vi "System Timing Test.vi"() -> ()   [LabVIEW 2020]
uses:
  e41e6262-df0e-46e3-b5d9-5448b0aad18a.vi
  71bacbc6-81ed-4225-8d97-44bb9760859f.vi
  57dc439b-a836-43f6-a4ee-51e2563579e4.vi
  <vilib>/Utility/High Resolution Relative Seconds.vi
  <vilib>/Analysis/NI_AALPro.lvlib
  <vilib>/gmath/NI_Gmath.lvlib
panel:
  out "Waveform Graph":dbl[](graph)
  out "median 3":dbl format="%.3f ms"
  out "timing 3":T1(graph)
  out "median 2":dbl format="%.3f ms"
  out "timing 2":T1(graph)
  out "median":dbl format="%.3f ms"
  out "timing":T1(graph)
  in  "repeats":i32=1800
  in  "milliseconds to wait":u32=990
  out "Iteration":i32
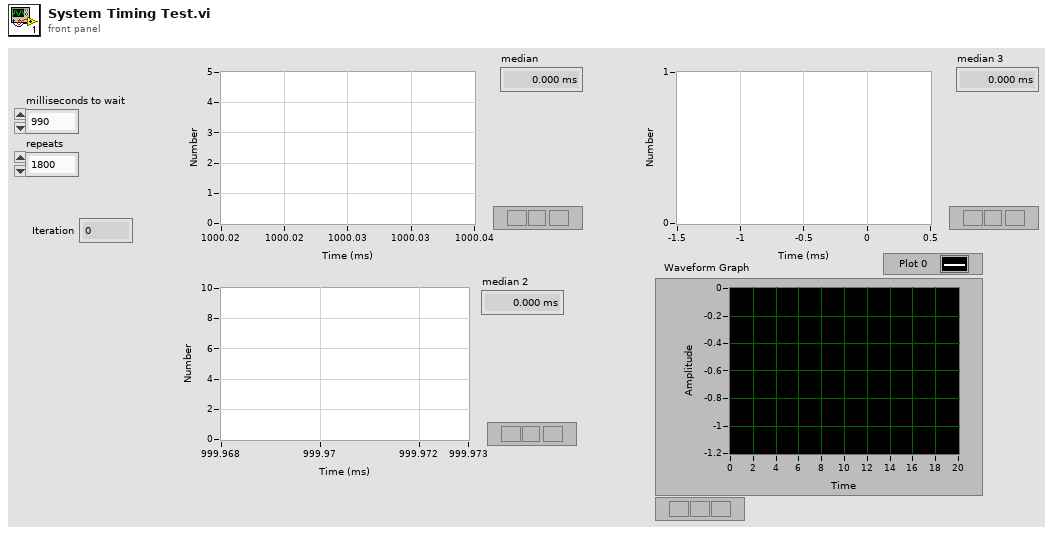
[diagram p1: front panel]
types:
  T1 = cluster{"X Values":dbl[], "Histogram: h(x)":i32[]}
  T2 = enum16{"arithmetic", "geometric", "harmonic", "trimmed", "median"}
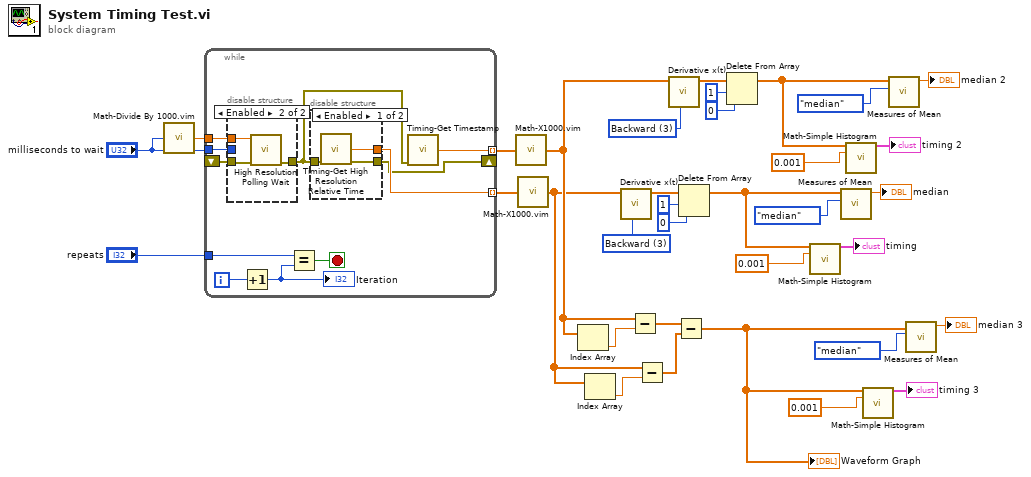
[diagram p0: block diagram]
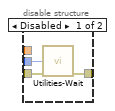
[diagram p2: hidden frame]
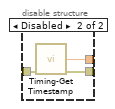
[diagram p3: hidden frame]
diagram:
  w20 = u16 3 items=["2nd Order Central", "4th Order Central", "Forward", "Backward"] ("method")
  w32 = u16 3 items=["2nd Order Central", "4th Order Central", "Forward", "Backward"] ("method")
  n1 = call "Math-Divide By 1000.vim"("X"="milliseconds to wait") -> ("1000X"=w25:dbl)
  n2 = while {
    tunnel: "repeats" -> [w45]
    tunnel: "milliseconds to wait" -> [w44]
    shift-right: [w36] -> _
    shift-left: _ -> [w42]
    tunnel: [w41] -> w33 mode=indexing
    tunnel: w25 -> [w38]
    tunnel: [w37] -> w21 mode=indexing
    i -> [w40]
    stop <- w43 stop-if-true
    n3 = disable-structure shown="Enabled" {
      disable-tunnel: w44 -> [w48 _]
      disable-tunnel: [w47 w50] -> w35
      disable-tunnel: w42 -> [w46 w51]
      disable-tunnel: w38 -> [_ w49]
      frame Disabled {
        n4 = call "Utilities-Wait.vi"("milliseconds to wait"=w48, "error in (no error)"=w46) -> ("error out"=w47:errorcluster)  [unwired: 13 in]
      }
      frame Enabled {
        n5 = call <vilib>:"High Resolution Polling Wait.vi"("error in (no error)"=w51, "seconds to wait"=w49) -> ("error out"=w50:errorcluster)  [unwired: 9 in]
      }
    }
    n6 = Increment(x=w40) -> (x+1=w39:i32)
    "Iteration" <- w39
    n7 = Equal?(x=w45, y=w39) -> (x = y?=w43:bool)
    n8 = disable-structure shown="Enabled" {
      disable-tunnel: w35 -> [w54 w57]
      disable-tunnel: [w53 w56] -> w36
      disable-tunnel: [w52 w55] -> w41
      frame Enabled {
        n9 = call "Timing-Get High Resolution Relative Time.vi"("error in (no error)"=w54) -> ("double precision float"=w52:dbl, "error out"=w53:errorcluster)  [unwired: 13 in]
      }
      frame Disabled {
        n10 = call "Timing-Get Timestamp.vi"("error in (no error)"=w57) -> ("double precision float"=w55:dbl, "error out"=w56:errorcluster)  [unwired: 13 in]
      }
    }
    n11 = call "Timing-Get Timestamp.vi"("error in (no error)"=w35) -> ("double precision float"=w37:dbl)  [unwired: 13 in, 1 out]
  }
  n12 = call "Math-X1000.vim"("X"=w21) -> ("1000X"=w6:dbl[])
  n13 = call "Math-X1000.vim"("X"=w33) -> ("1000X"=w2:dbl[])
  n14 = Index Array(array=w6) -> (element=w7:dbl)  [unwired: 1 in]
  n15 = Index Array(array=w2) -> (element=w4:dbl)  [unwired: 1 in]
  n16 = call <vilib>:"Derivative x(t).vi"("method"=w32, "X"=w2) -> ("dX/dt"=w31:dbl[])  [unwired: 8 in, 1 out]
  n17 = Subtract(x=w6, y=w7) -> (x-y=w5:dbl[])
  n18 = Subtract(x=w2, y=w4) -> (x-y=w3:dbl[])
  n19 = call <vilib>:"Derivative x(t).vi"("method"=w20, "X"=w6) -> ("dX/dt"=w19:dbl[])  [unwired: 8 in, 1 out]
  n20 = Subtract(x=w5, y=w3) -> (x-y=w1:dbl[])
  "Waveform Graph" <- w1
  n21 = Delete From Array(array=w31, length=1, index=0) -> (array with subset deleted=w24:dbl[])  [unwired: 1 out]
  n22 = Delete From Array(array=w19, length=1, index=0) -> (array with subset deleted=w14:dbl[])  [unwired: 1 out]
  n23 = call "Math-Simple Histogram.vi"("Array"=w24, "Binwidth"=0.001 ("Step")) -> ("Histogram Graph"=→"timing":T1)  [unwired: 13 in]
  n24 = call <vilib>:"Measures of Mean.vi"("type"=T2."median", "x array"=w24) -> ("mean value"=→"median":dbl)  [unwired: 8 in, 1 out]
  n25 = call "Math-Simple Histogram.vi"("Array"=w14, "Binwidth"=0.001 ("Step")) -> ("Histogram Graph"=→"timing 2":T1)  [unwired: 13 in]
  n26 = call "Math-Simple Histogram.vi"("Array"=w1, "Binwidth"=0.001 ("Step")) -> ("Histogram Graph"=→"timing 3":T1)  [unwired: 13 in]
  n27 = call <vilib>:"Measures of Mean.vi"("type"=T2."median", "x array"=w14) -> ("mean value"=→"median 2":dbl)  [unwired: 8 in, 1 out]
  n28 = call <vilib>:"Measures of Mean.vi"("type"=T2."median", "x array"=w1) -> ("mean value"=→"median 3":dbl)  [unwired: 8 in, 1 out]
